vi "RT__only_FIFO_healty.vi"(8 "error in (no error)":errorcluster) -> (0 "error out":errorcluster, 3 "output cluster":T1)   [LabVIEW 2020]
uses:
  RT_only_FIFO_Health.ctl
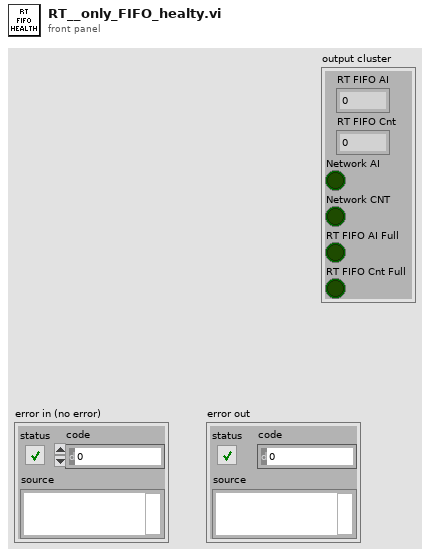
[diagram p1: front panel]
types:
  T1 = typedef "RT_only_FIFO_Health.ctl" = cluster{"RT FIFO AI":i32, "RT FIFO Cnt":i32, "Network AI":bool, "Network CNT":bool, "RT FIFO AI Full":bool, "RT FIFO Cnt Full":bool}
  T2 = cluster{"Int32":i32, "Int32":i32, "Boolean":bool, "Boolean":bool, "Boolean":bool, "Boolean":bool}
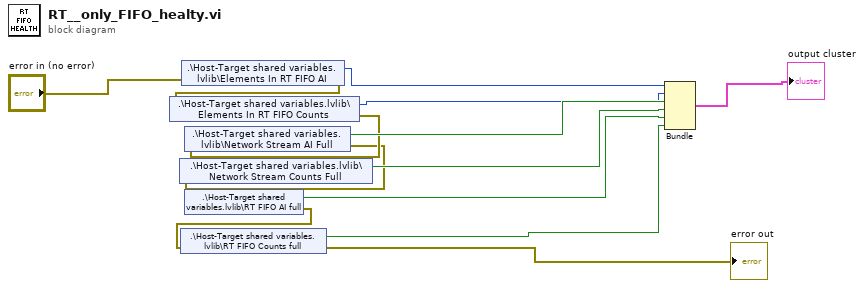
[diagram p0: block diagram]
diagram:
  n1 = shared-variable ".\\Host-Target shared variables.lvlib\\Elements In RT FIFO AI"(error in="error in (no error)") -> (w8:i32, error out=w5:errorcluster)
  n2 = shared-variable ".\\Host-Target shared variables.lvlib\\Elements In RT FIFO Counts"(error in=w5) -> (w9:i32, error out=w4:errorcluster)
  n3 = shared-variable ".\\Host-Target shared variables.lvlib\\Network Stream AI Full"(error in=w4) -> (w10:bool, error out=w3:errorcluster)
  n4 = shared-variable ".\\Host-Target shared variables.lvlib\\Network Stream Counts Full"(error in=w3) -> (w11:bool)  [unwired: 1 out]
  n5 = shared-variable ".\\Host-Target shared variables.lvlib\\RT FIFO AI full"() -> (w12:bool, error out=w2:errorcluster)  [unwired: 1 in]
  n6 = shared-variable ".\\Host-Target shared variables.lvlib\\RT FIFO Counts full"(error in=w2) -> (w13:bool, error out=→"error out":errorcluster)
  n7 = Bundle("Int32"=w8, "Int32"=w9, "Boolean"=w10, "Boolean"=w11, "Boolean"=w12, "Boolean"=w13) -> (→"output cluster":T2)  [unwired: 1 in]
